vi "数据插入.vi"(5 "数据标记表":string(combo)="N", 7 "测量模式":string(combo), 8 "error in (no error)":errorcluster caption="错误输入（无错误）", 10 "data in":T1={"因子编码"="", "单位"="", "标样参考值"=0.0, "水样数据时间"=timestamp(0 s since 1904-01-01), "水样实测值"=0.0, "水样数据标识"="N", "探头温度"=0.0}, 11 "table输入":string(combo)) -> (0 "error out":errorcluster caption="错误输出")   [LabVIEW 2016, in "斯坦道多参数.lvlib"]
uses:
  <vilib>/Utility/sysdir.llb/System Directory Type.ctl
  <vilib>/Utility/error.llb/DialogType.ctl
  <vilib>/addons/database/Connection.llb/DB Tools Open Connec (String).vi
  <vilib>/addons/database/Connection.llb/Conn Execute.vi
  <vilib>/addons/database/Recordset.llb/Rec Destroy - Connection.vi
  <vilib>/addons/database/NI_Database_API.lvlib
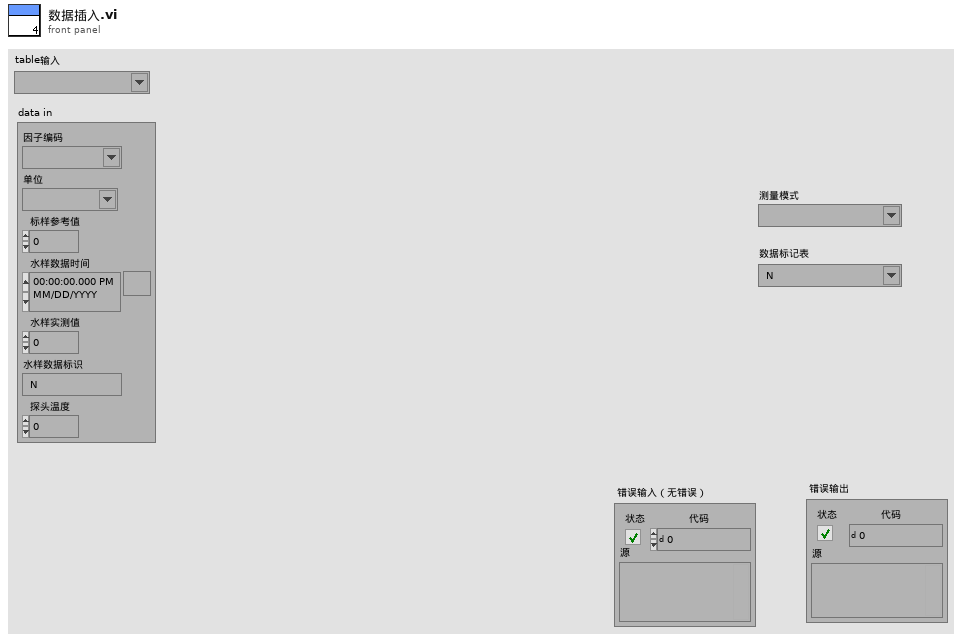
[diagram p1: front panel]
types:
  T1 = cluster{"因子编码":string, "单位":string, "标样参考值":sgl, "水样数据时间":timestamp, "水样实测值":sgl, "水样数据标识":string, "探头温度":sgl}
  T2 = typedef "DialogType.ctl" = u16
  T3 = typedef "System Directory Type.ctl" = i32
  T4 = cluster{"时间标识":timestamp, "测量模式":string, "数据类型":string, "监测值":sgl, "单位":string, "数据标识":string, "因子编码":string, "标样参考值":sgl, "探头温度":sgl, "LastTime":timestamp}
  T5 = typedef "NI_Database_API.lvlib/Conn ObjectReference.ctl" = refnum<k1>
  T6 = typedef "NI_Database_API.lvlib/Rec ObjectReference.ctl" = refnum<k1>
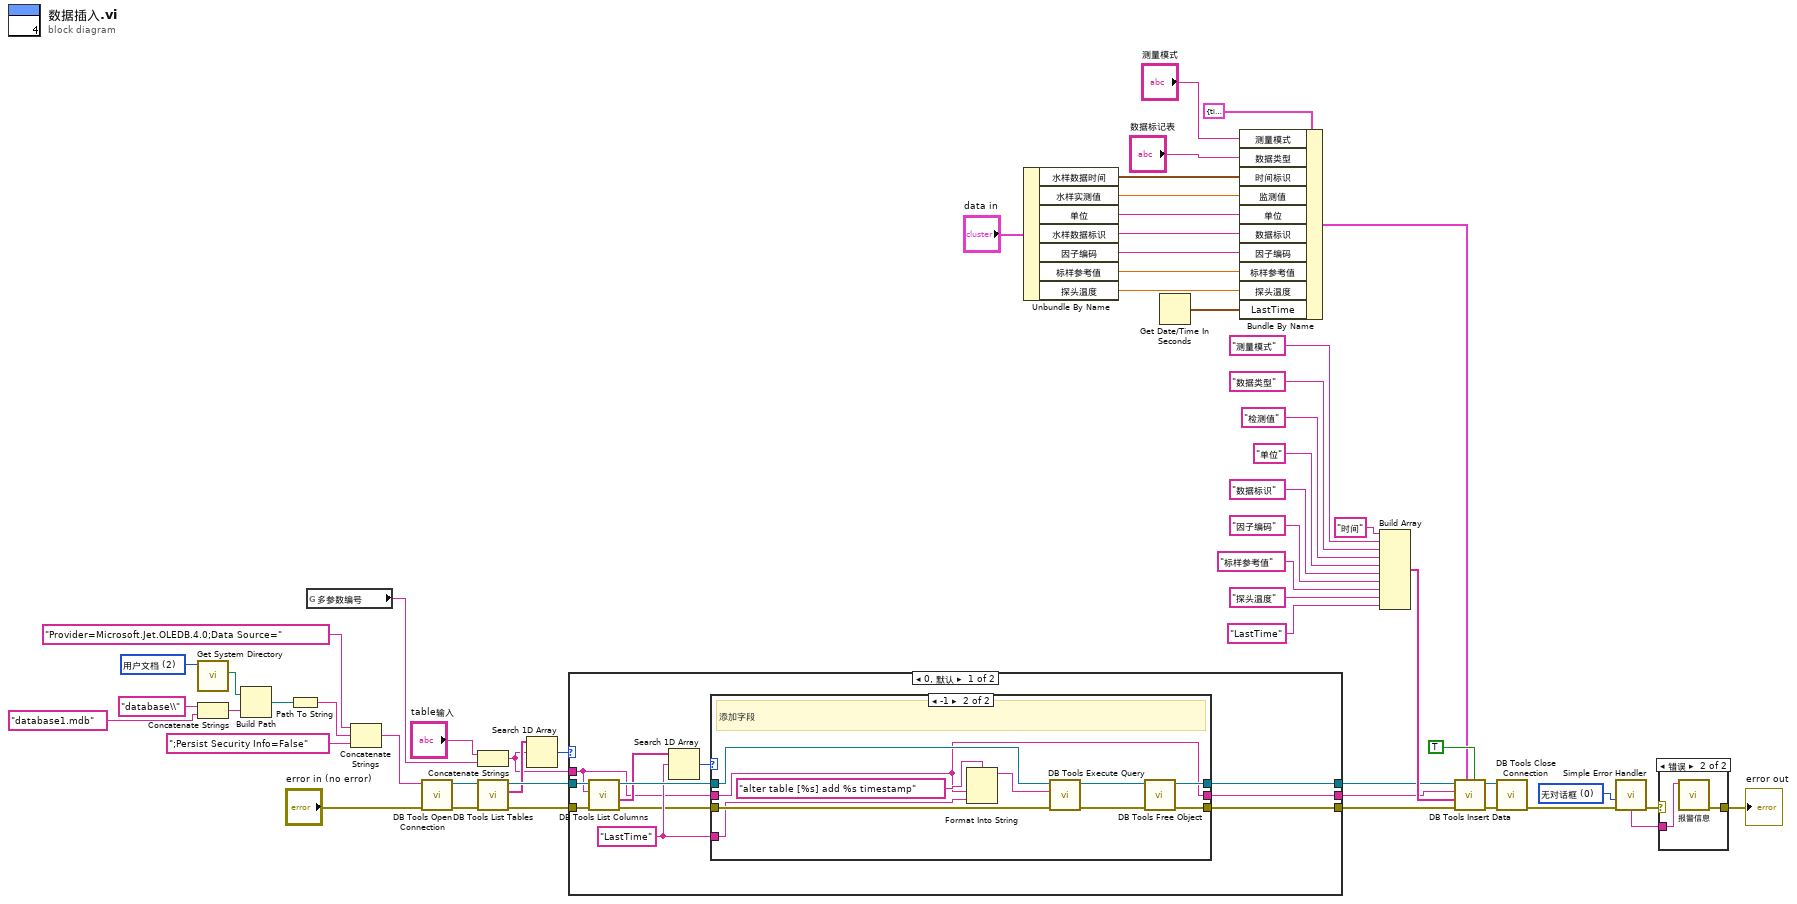
[diagram p0: block diagram]
diagram:
  w12 = T2 0 items=["无对话框", "确定信息", "继续或停止信息", "确定信息＋警告", "继续/停止+警告"] ("type of dialog (OK msg:1)")
  w36 = T3 2 items=["用户目录"=0, "用户桌面"=1, "用户文档"=2, "用户应用程序数据"=3, "用户设置"=4, "用户临时目录"=5, "公共文档"=6, "公共应用程序数据"=7, "公共设置"=8, "公共缓存"=13, "系统核心库"=9, "系统安装库"=10, "应用程序文件"=11, "启动盘根目录"=12] ("system directory type")
  n1 = call <vilib>:"Get System Directory.vi"("system directory type"=w36) -> ("system directory"=w34:path)  [unwired: 10 in]
  n2 = Concatenate Strings("database\\" ("condition"), "database1.mdb" ("字符串")) -> (w28:string)
  n3 = Build Path(base path=w34, name or relative path=w28) -> (appended path=w33:path)
  n4 = Path To String(path=w33) -> (string=w32:string)
  n5 = global read "多参数全局变量.vi" "多参数编号"() -> (w1:string)
  n6 = Concatenate Strings("Provider=Microsoft.Jet.OLEDB.4.0;Data Source=" ("condition"), w32, ";Persist Security Info=False" ("condition")) -> (w30:string)
  n7 = call-poly <vilib>:"DB Tools Open Connection.vi"("error in (no error)"="error in (no error)", "connection information"=w30) -> ("error out"=w7:errorcluster, "connection reference"=w20:T5)  [unwired: 6 in]
  n8 = Concatenate Strings("table输入", w1) -> (w2:string)
  n9 = call <vilib>:"DB Tools List Tables.vi"("error in (no error)"=w7, "connection reference"=w20) -> ("error out"=w6:errorcluster, "tables"=w5:string[], "connection reference out"=w8:T5)  [unwired: 3 in]
  n10 = Search 1D Array(1D array=w5, element=w2) -> (index of element=w3:i32)  [unwired: 1 in]
  n11 = case shown="0, 默认" w3 {
    tunnel: [w61 w82] -> w19
    tunnel: [w60 w80] -> w18
    tunnel: [w59 w81] -> w17
    tunnel: w8 -> [w58 w82]
    tunnel: w6 -> [w57 w80]
    tunnel: w2 -> [w56 w81]
    frame 0, Default {
      w65 = "LastTime" ("元素")
      n12 = call <vilib>:"DB Tools List Columns.vi"("error in (no error)"=w57, "table"=w56, "connection reference"=w58) -> ("error out"=w63:errorcluster, "columns"=w64:string[], "connection reference out"=w66:T5)  [unwired: 1 in, 1 out]
      n13 = Search 1D Array(1D array=w64, element=w65) -> (index of element=w62:i32)  [unwired: 1 in]
      n14 = case shown="-1" w62 {
        tunnel: w66 -> [w69 w77]
        tunnel: w63 -> [w68 w76]
        tunnel: w65 -> [_ w74]
        tunnel: [w69 w72] -> w61
        tunnel: [w68 w71] -> w60
        tunnel: w56 -> [w67 w70]
        tunnel: [w67 w70] -> w59
        frame 0, Default {
        }
        frame -1 {
          # "添加字段"
          n15 = Format Into String(format string="alter table [%s] add %s timestamp", w70, w74) -> (resulting string=w73:string)  [unwired: 2 in, 1 out]
          n16 = call-poly <vilib>:"DB Tools Execute Query.vi"("error in (no error)"=w76, "SQL query"=w73, "connection reference"=w77) -> ("error out"=w78:errorcluster, "recordset reference"=w79:T6)  [unwired: 5 in]
          n17 = call-poly <vilib>:"DB Tools Free Object.vi"("error in (no error)"=w78, "recordset reference"=w79) -> ("error out"=w71:errorcluster, "connection reference"=w72:T5)  [unwired: 8 in]
        }
      }
    }
    frame -1 {
    }
  }
  n18 = Unbundle By Name("data in") -> ("水样数据时间"=w50:timestamp, "水样实测值"=w49:sgl, "单位"=w45:string, "水样数据标识"=w48:string, "因子编码"=w44:string, "标样参考值"=w46:sgl, "探头温度"=w25:sgl)
  n19 = Get Date/Time In Seconds() -> (seconds since 1Jan1904=w15:timestamp)
  n20 = Bundle By Name(cluster=T4 {"时间标识"=timestamp(0 s since 1904-01-01), "测量模式"="", "数据类型"="", "监测值"=0.0, "单位"="", "数据标识"="", "因子编码"="", "标样参考值"=0.0, "探头温度"=0.0, "LastTime"=timestamp(0 s since 1904-01-01)} ("data输出"), "测量模式"="测量模式", "数据类型"="数据标记表", "时间标识"=w50, "监测值"=w49, "单位"=w45, "数据标识"=w48, "因子编码"=w44, "标样参考值"=w46, "探头温度"=w25, "LastTime"=w15) -> (w26:T4)
  n21 = Build Array("时间", "测量模式", "数据类型", "检测值", "单位", "数据标识", "因子编码", "标样参考值", "探头温度", "LastTime") -> (w27:string[])
  n22 = call <vilib>:"DB Tools Insert Data.vi"("create table? (F)"=TRUE, "data"=w26, "error in (no error)"=w18, "columns"=w27, "table"=w17, "connection reference"=w19) -> ("error out"=w38:errorcluster, "connection reference out"=w39:T5)  [unwired: 4 in]
  n23 = call <vilib>:"DB Tools Close Connection.vi"("error in (no error)"=w38, "connection reference"=w39) -> ("error out"=w13:errorcluster)  [unwired: 5 in]
  n24 = call <vilib>:"Simple Error Handler.vi"("type of dialog (OK msg:1)"=w12, "error in (no error)"=w13) -> ("error out"=w10:errorcluster, "message"=w11:string)  [unwired: 3 in, 3 out]
  n25 = case shown="错误" w10 {
    selector: w10 -> [w83 _]
    tunnel: w11 -> [_ w85]
    tunnel: [w83 w84] -> w9
    frame No Error {
    }
    frame Error {
      n26 = call "报警信息.vi"("报警信息"=w85) -> ("error out"=w84:errorcluster)  [unwired: 10 in]
    }
  }
  "error out" <- w9
